vi "C alpha to the power n.vi"(1 "alpha":dbl=0.5, 2 "c":dbl=1.0, 3 "n":i32=128) -> (0 "Waveform Graph":dbl[](graph)=[1.0, 0.5, 0.25, 0.125, 0.0625, 0.03125, 0.015625, 0.0078125, 0.00390625, 0.001953125, 0.0009765625, 0.00048828125, 0.000244140625, 0.0001220703125, 6.103515625e-05, 3.0517578125e-05, 1.52587890625e-05, 7.62939453125e-06, 3.814697265625e-06, 1.9073486328125e-06, 9.5367431640625e-07, 4.76837158203125e-07, 2.384185791015625e-07, 1.1920928955078125e-07, 5.960464477539063e-08, 2.9802322387695312e-08, 1.4901161193847656e-08, 7.450580596923828e-09, 3.725290298461914e-09, 1.862645149230957e-09, 9.313225746154785e-10, 4.656612873077393e-10, 2.3283064365386963e-10, 1.1641532182693481e-10, 5.820766091346741e-11, 2.9103830456733704e-11, 1.4551915228366852e-11, 7.275957614183426e-12, 3.637978807091713e-12, 1.8189894035458565e-12, 9.094947017729282e-13, 4.547473508864641e-13, 2.2737367544323206e-13, 1.1368683772161603e-13, 5.684341886080802e-14, 2.842170943040401e-14, 1.4210854715202004e-14, 7.105427357601002e-15, 3.552713678800501e-15, 1.7763568394002505e-15, 8.881784197001252e-16, 4.440892098500626e-16, 2.220446049250313e-16, 1.1102230246251565e-16, 5.551115123125783e-17, 2.7755575615628914e-17, 1.3877787807814457e-17, 6.938893903907228e-18, 3.469446951953614e-18, 1.734723475976807e-18, 8.673617379884035e-19, 4.336808689942018e-19, 2.168404344971009e-19, 1.0842021724855044e-19, 5.421010862427522e-20, 2.710505431213761e-20, 1.3552527156068805e-20, 6.776263578034403e-21, 3.3881317890172014e-21, 1.6940658945086007e-21, 8.470329472543003e-22, 4.235164736271502e-22, 2.117582368135751e-22, 1.0587911840678754e-22, 5.293955920339377e-23, 2.6469779601696886e-23, 1.3234889800848443e-23, 6.617444900424222e-24, 3.308722450212111e-24, 1.6543612251060553e-24, 8.271806125530277e-25, 4.1359030627651384e-25, 2.0679515313825692e-25, 1.0339757656912846e-25, 5.169878828456423e-26, 2.5849394142282115e-26, 1.2924697071141057e-26, 6.462348535570529e-27, 3.2311742677852644e-27, 1.6155871338926322e-27, 8.077935669463161e-28, 4.0389678347315804e-28, 2.0194839173657902e-28, 1.0097419586828951e-28, 5.048709793414476e-29, 2.524354896707238e-29, 1.262177448353619e-29, 6.310887241768095e-30, 3.1554436208840472e-30, 1.5777218104420236e-30, 7.888609052210118e-31, 3.944304526105059e-31, 1.9721522630525295e-31, 9.860761315262648e-32, 4.930380657631324e-32, 2.465190328815662e-32, 1.232595164407831e-32, 6.162975822039155e-33, 3.0814879110195774e-33, 1.5407439555097887e-33, 7.703719777548943e-34, 3.851859888774472e-34, 1.925929944387236e-34, 9.62964972193618e-35, 4.81482486096809e-35, 2.407412430484045e-35, 1.2037062152420224e-35, 6.018531076210112e-36, 3.009265538105056e-36, 1.504632769052528e-36, 7.52316384526264e-37, 3.76158192263132e-37, 1.88079096131566e-37, 9.4039548065783e-38, 4.70197740328915e-38, 2.350988701644575e-38, 1.1754943508222875e-38, 5.877471754111438e-39])   [LabVIEW 2009]
doc: "This VI creates an array of n sample sequence given by the equation\nx[n] = C*alpha^n."
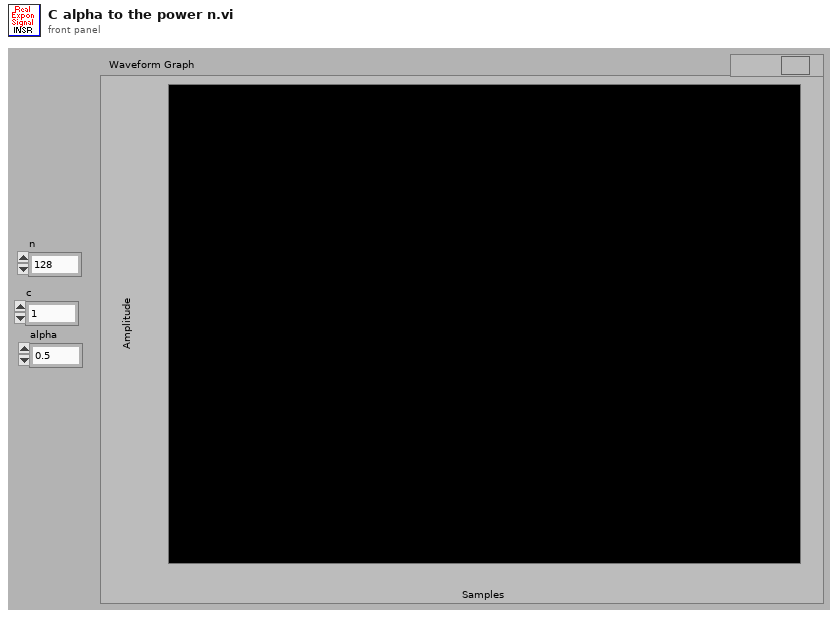
[diagram p1: front panel]
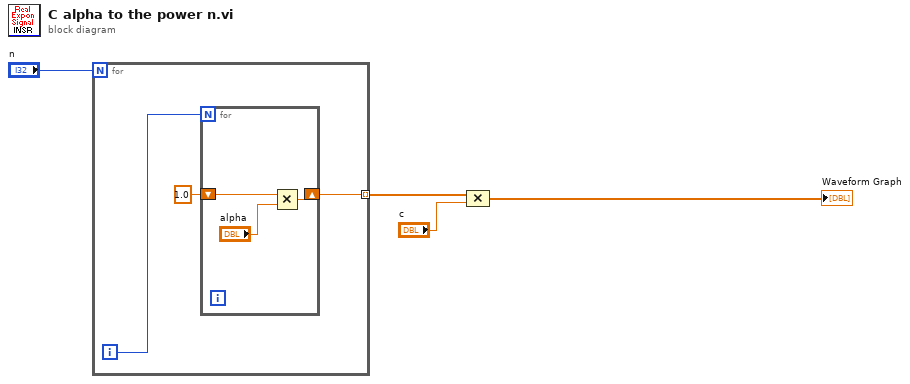
[diagram p0: block diagram]
diagram:
  n1 = for {
    N: "n" -> [_]
    tunnel: [w5] -> w3 mode=indexing
    i -> [w6]
    n2 = for {
      N: w6 -> [_]
      shift-right: [w9] -> w5
      shift-left: 1.0 -> [w8]
      n3 = Multiply(x=w8, y="alpha") -> (x*y=w9:dbl)
    }
  }
  n4 = Compound Arithmetic op=MULTIPLY(w3, "c") -> (→"Waveform Graph":dbl[])
